vi "IT7800 Driver commands.vi"(6 "Read":bool=TRUE, 7 "Command":T1, 8 "error in":errorcluster, 10 "Data Write":dbl, 11 "VISA in":refnum<visa-resource-name>="TCPIP::192.168.0.252::INSTR") -> (0 "error out":errorcluster, 1 "Data ASCII":string, 2 "Data Read":dbl, 3 "VISA out":refnum<visa-resource-name>)   [LabVIEW 2025]
uses:
  TypeDefs/CMD - Control.ctl
  <vilib>/Utility/error.llb/Trim Whitespace One-Sided.vi
  <instrlib>/IT7800/IT7800.lvlib
panel:
  # "\"Phases\" valid input:\n1=ONE(1)\n3=THRee(3)\n4=DIFFerence(reverse)\n5=MULTichannel\nNote: with small PSUs we use ONE & Reverse\nChange only when output OFF, reset Voltage\nafter change"
  # "\"Measure Rate\" valid input\n0=Fast (150ms)\n1=MEDium (300ms)\n2=SLOW (500ms)\n3=LOWer (1000ms)\n4=LOWest (1Hz)"
  # "IP7800 Driver V0.11\nDriver commands"
  # "19.05.2025"
  # "Andrej Valand"
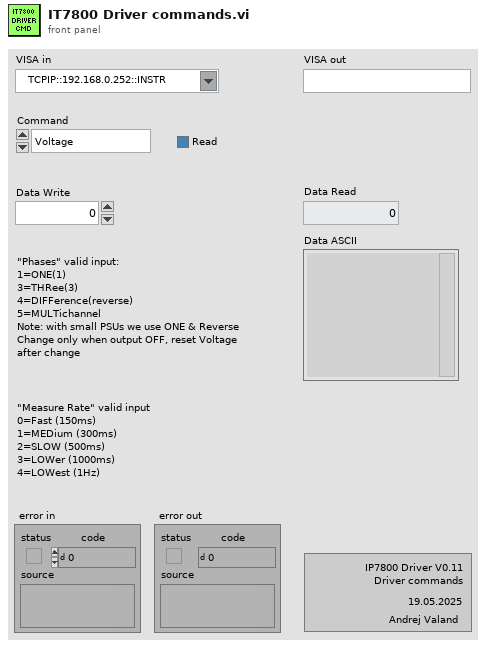
[diagram p1: front panel]
types:
  T1 = typedef "CMD - Control.ctl" = enum16{"Voltage", "Frquency", "Set Phases", "Output", "Measure Rate"}
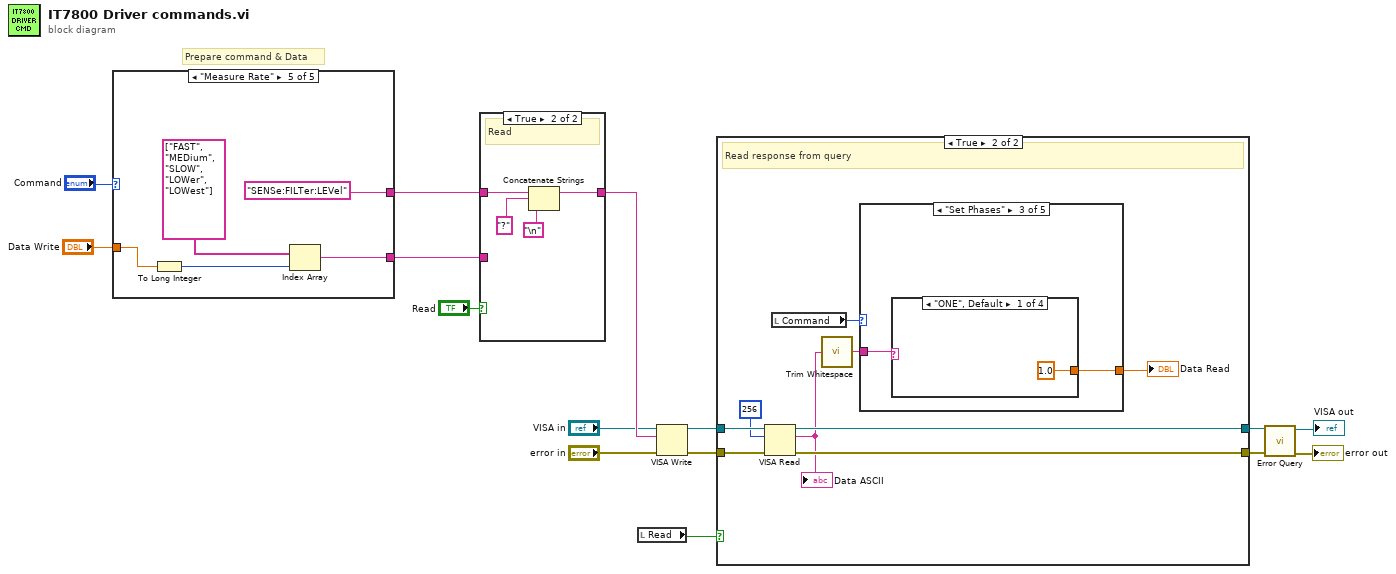
[diagram p0: block diagram]
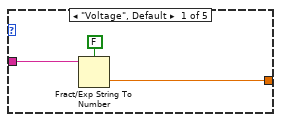
[diagram p3: hidden frame]
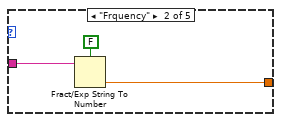
[diagram p4: hidden frame]
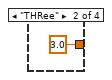
[diagram p5: hidden frame]
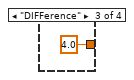
[diagram p6: hidden frame]
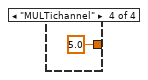
[diagram p7: hidden frame]
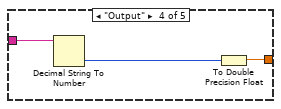
[diagram p8: hidden frame]
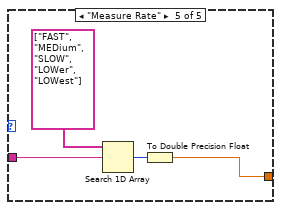
[diagram p9: hidden frame]
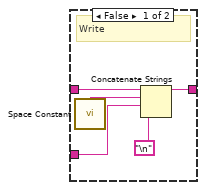
[diagram p10: hidden frame]
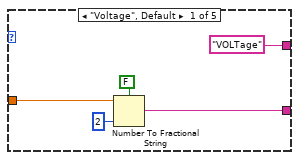
[diagram p11: hidden frame]
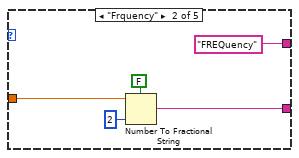
[diagram p12: hidden frame]
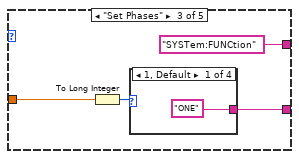
[diagram p13: hidden frame]
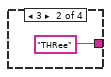
[diagram p14: hidden frame]
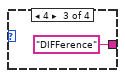
[diagram p15: hidden frame]
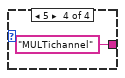
[diagram p16: hidden frame]
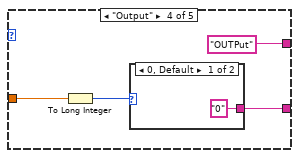
[diagram p17: hidden frame]
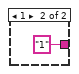
[diagram p18: hidden frame]
diagram:
  # "Prepare command & Data"
  n1 = case shown="\"Measure Rate\"" "Command" {
    tunnel: ["VOLTage" "FREQuency" "SYSTem:FUNCtion" "OUTPut" "SENSe:FILTer:LEVel"] -> w13
    tunnel: "Data Write" -> [w19 w22 w28 w36 w43]
    tunnel: [w16 w21 w26 w34 w40] -> w5
    frame "Voltage", Default {
      n2 = Number To Fractional String(use system decimal point (T)=FALSE, number=w19, precision (6)=i16 2) -> (F-format string=w16:string)  [unwired: 1 in]
    }
    frame "Frquency" {
      n3 = Number To Fractional String(use system decimal point (T)=FALSE, number=w22, precision (6)=i16 2) -> (F-format string=w21:string)  [unwired: 1 in]
    }
    frame "Set Phases" {
      n4 = To Long Integer(number=w28) -> (32bit integer=w27:i32)
      n5 = case shown="1, Default" w27 {
        tunnel: ["ONE" "THRee" "DIFFerence" "MULTichannel"] -> w26
        frame 1, Default {
        }
        frame 3 {
        }
        frame 4 {
        }
        frame 5 {
        }
      }
    }
    frame "Output" {
      n6 = To Long Integer(number=w36) -> (32bit integer=w35:i32)
      n7 = case shown="0, Default" w35 {
        tunnel: ["0" "1"] -> w34
        frame 0, Default {
        }
        frame 1 {
        }
      }
    }
    frame "Measure Rate" {
      n8 = To Long Integer(number=w43) -> (32bit integer=w41:i32)
      n9 = Index Array(array=string[] ["FAST", "MEDium", "SLOW", "LOWer", "LOWest"], index=w41) -> (element=w40:string)
    }
  }
  n10 = case shown="True" "Read" {
    tunnel: w13 -> [w49 w53]
    tunnel: [w48 w51] -> w10
    tunnel: w5 -> [w46 _]
    frame False {
      # "Write"
      n11 = call <vilib>:"Space Constant.vi"() -> ("String"=w45:string)
      n12 = Concatenate Strings(w49, w45, w46, "\n") -> (w48:string)
    }
    frame True {
      # "Read"
      n13 = Concatenate Strings(w53, "?", "\n") -> (w51:string)
    }
  }
  n14 = local read "Read"() -> (w7:bool)
  n15 = VISA Write(VISA resource name="VISA in", write buffer=w10, error in (no error)="error in") -> (VISA resource name out=w12:refnum<visa-resource-name>, error out=w11:errorcluster)  [unwired: 1 out]
  n16 = case shown="True" w7 {
    tunnel: w12 -> [w55 w64]
    tunnel: w11 -> [w54 w63]
    tunnel: [w55 w60] -> w4
    tunnel: [w54 w59] -> w2
    frame False {
      # "Instruments returns nothing on writes"
    }
    frame True {
      # "Read response from query"
      n17 = VISA Read(VISA resource name=w64, byte count=u32 256, error in (no error)=w63) -> (VISA resource name out=w60:refnum<visa-resource-name>, read buffer=w56:string, error out=w59:errorcluster)  [unwired: 1 out]
      "Data ASCII" <- w56
      n18 = local read "Command"() -> (w61:T1)
      n19 = call <vilib>:"Trim Whitespace.vi"("string"=w56) -> ("trimmed string"=w57:string)  [unwired: 1 in]
      n20 = case shown="\"Set Phases\"" w61 {
        tunnel: w57 -> [w67 w69 w72 w79 w82]
        tunnel: [w65 w68 w71 w78 w80] -> w58
        frame "Voltage", Default {
          n21 = Fract/Exp String To Number(use system decimal point (T)=FALSE, string=w67) -> (number=w65:dbl)  [unwired: 2 in, 1 out]
        }
        frame "Frquency" {
          n22 = Fract/Exp String To Number(use system decimal point (T)=FALSE, string=w69) -> (number=w68:dbl)  [unwired: 2 in, 1 out]
        }
        frame "Set Phases" {
          n23 = case shown="\"ONE\", Default" w72 {
            tunnel: [1.0 3.0 4.0 5.0] -> w71
            frame "ONE", Default {
            }
            frame "THRee" {
            }
            frame "DIFFerence" {
            }
            frame "MULTichannel" {
            }
          }
        }
        frame "Output" {
          n24 = Decimal String To Number(string=w79) -> (number=w77:i32)  [unwired: 2 in, 1 out]
          n25 = To Double Precision Float(number=w77) -> (double precision float=w78:dbl)
        }
        frame "Measure Rate" {
          n26 = Search 1D Array(1D array=string[] ["FAST", "MEDium", "SLOW", "LOWer", "LOWest"], element=w82) -> (index of element=w81:i32)  [unwired: 1 in]
          n27 = To Double Precision Float(number=w81) -> (double precision float=w80:dbl)
        }
      }
      "Data Read" <- w58
    }
  }
  n28 = call <instrlib>:"Error Query.vi"("error in"=w2, "VISA resource name"=w4) -> ("error out"=→"error out":errorcluster, "VISA resource name out"=→"VISA out":refnum<visa-resource-name>)  [unwired: 6 in, 2 out]
